vi "Configure Waveform Function.vi"(8 "error in (no error)":errorcluster, 9 "Waveform Function (0: Sine)":u16(ring) items=["Sine", "Square", "Ramp", "DC", "Pulse", "Arb", "Noise", "PRBS", "IQ"], 10 "Channel (1:Channel 1)":i32(ring)=1 items=["Channel 1"=1, "Channel 2"=2], 11 "VISA resource name":refnum<visa-resource-name>) -> (0 "error out":errorcluster, 3 "VISA resource name out":refnum<visa-resource-name>)   [LabVIEW 2019, in "Siglent SDG X Series.lvlib"]
doc: "Configure the waveform that you want the function generator to produce."
uses:
  Siglent SDG X Series.lvlib
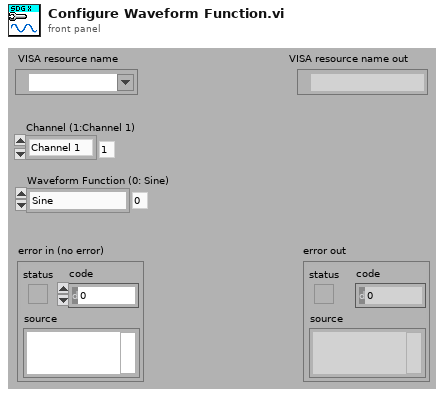
[diagram p1: front panel]
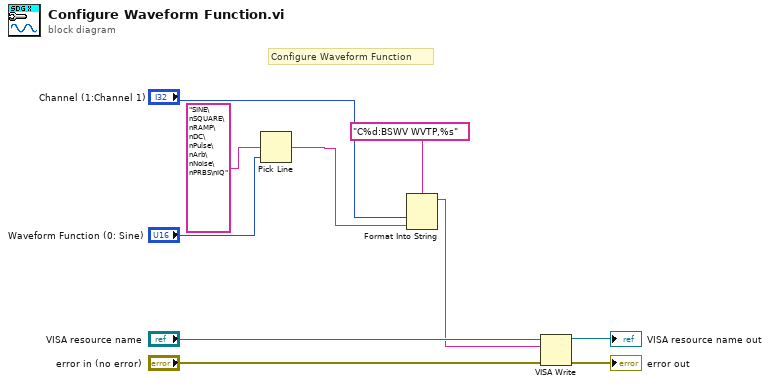
[diagram p0: block diagram]
diagram:
  # "Configure Waveform Function"
  n1 = Pick Line(multi-line string="SINE\nSQUARE\nRAMP\nDC\nPulse\nArb\nNoise\nPRBS\nIQ", line index="Waveform Function (0: Sine)") -> (output string=w9:string)  [unwired: 1 in]
  n2 = Format Into String(format string="C%d:BSWV WVTP,%s", "Channel (1:Channel 1)", w9) -> (resulting string=w6:string)  [unwired: 2 in, 1 out]
  n3 = VISA Write(VISA resource name="VISA resource name", write buffer=w6, error in (no error)="error in (no error)") -> (VISA resource name out=→"VISA resource name out":refnum<visa-resource-name>, error out=→"error out":errorcluster)  [unwired: 1 out]
